vi "Problem_01b.vi"() -> ()   [LabVIEW 2023]
uses:
  <vilib>/regexp/Match Regular Expression.xnode
panel:
  out "string array":string[](array[string])
  out "x = y?":bool[](array[boolean])
  out "Array 2":i32[](array[numeric])
  out "sum":i32
  out "Array":i32[](array[numeric])
  in  "Puzzle":string="9cbncbxclbvkmfzdnldc\njjn1drdffhs\n3six7\n38rgtnqqxtc\nrxszdkkv3j8kjhbm\n54nzzddht8ninelrkkseightseven6\n6fourmnvkgnthjtnjqkr\nnineninezsstmkone4sjnlbldcrj4eight\n3rdnfkvrx4twoqgeightqkgmn\n6mlhponeglrzrvbsseven\nfive8spgxz8\n3three2dfourfour58\n9q\ntwo45\nfive8mpkpdfiveeightfourseven\n93threefive3three92\n6jdzeightnineone1sclhzrnrjxfive\n6nseven16lbztpbbzthree8five\neight6mntljvbfrmftsffchsix4\n4twosixvnhjl\n8d\neightsevenvqvzlqxkbm6rqhsgqpnine7twonex\nseven96\nck8tv6\n2mcddqpnbxssmrc6\nzsfbkrjjqpbbone6six2\nfourone8hfrkxrr\n7ninetphdpcx\n9gcn9six4mfnjgtcdc\n6onevsevenseven4three\nldssggpknine7\ntwolltbfkhltwo892jngx\nrsh1f..."
  in  "Sample":string="two1nine\neightwothree\nabcone2threexyz\nxtwone3four\n4nineeightseven2\nzoneight234\n7pqrstsixteen"
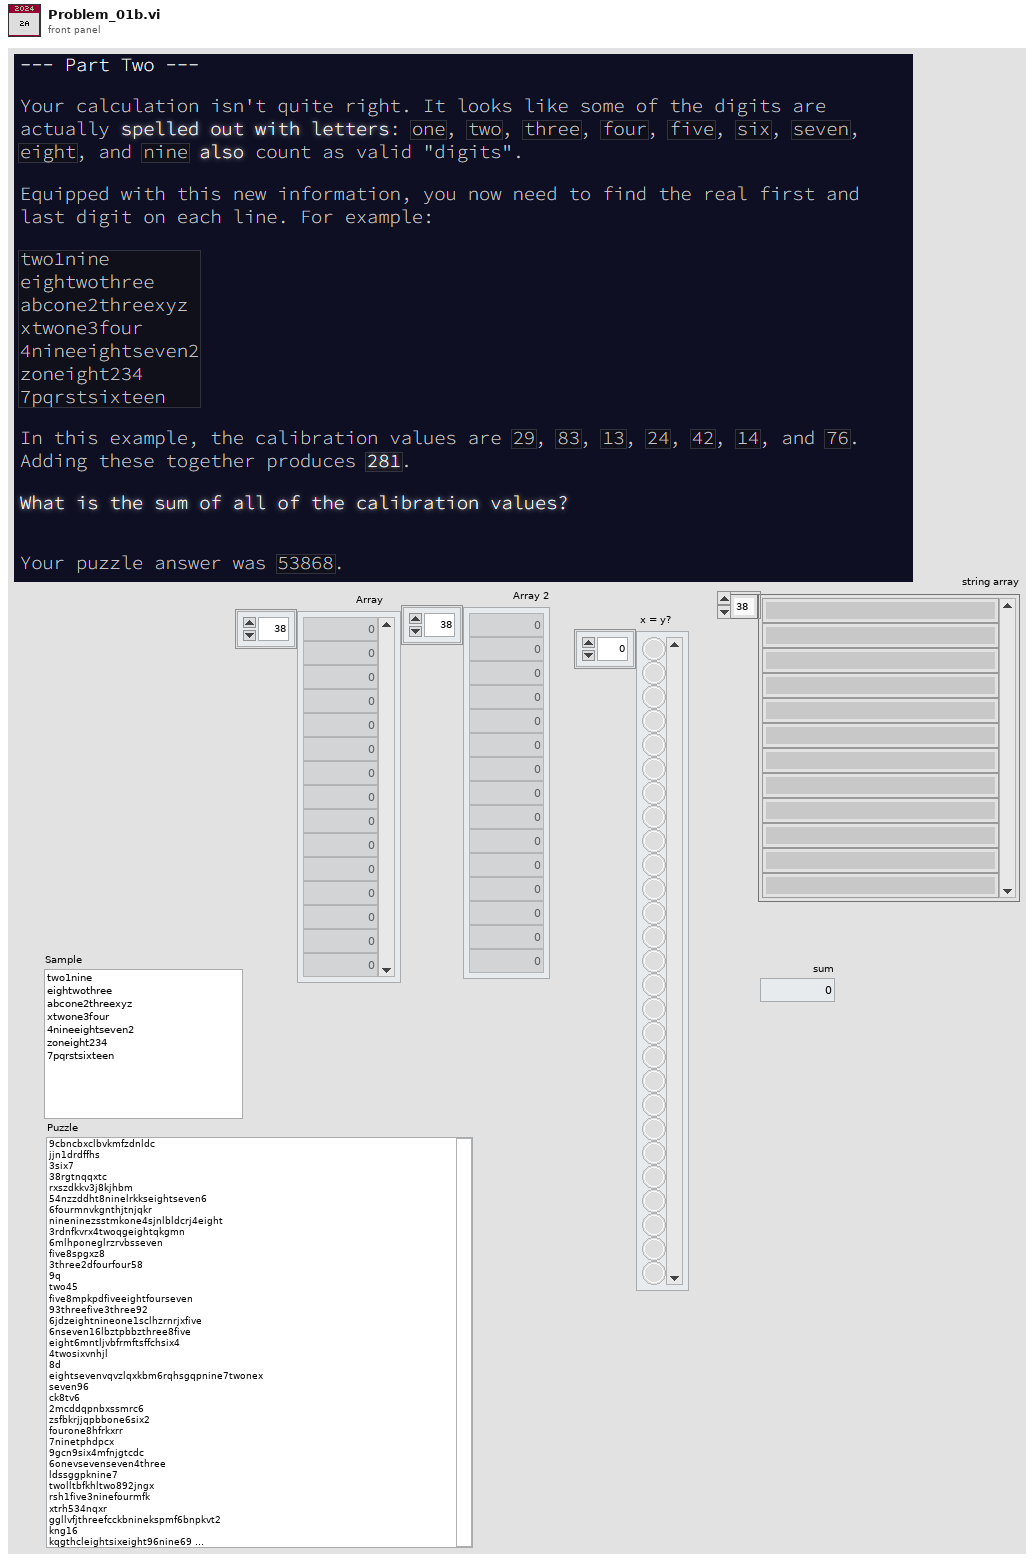
[diagram p1: front panel]
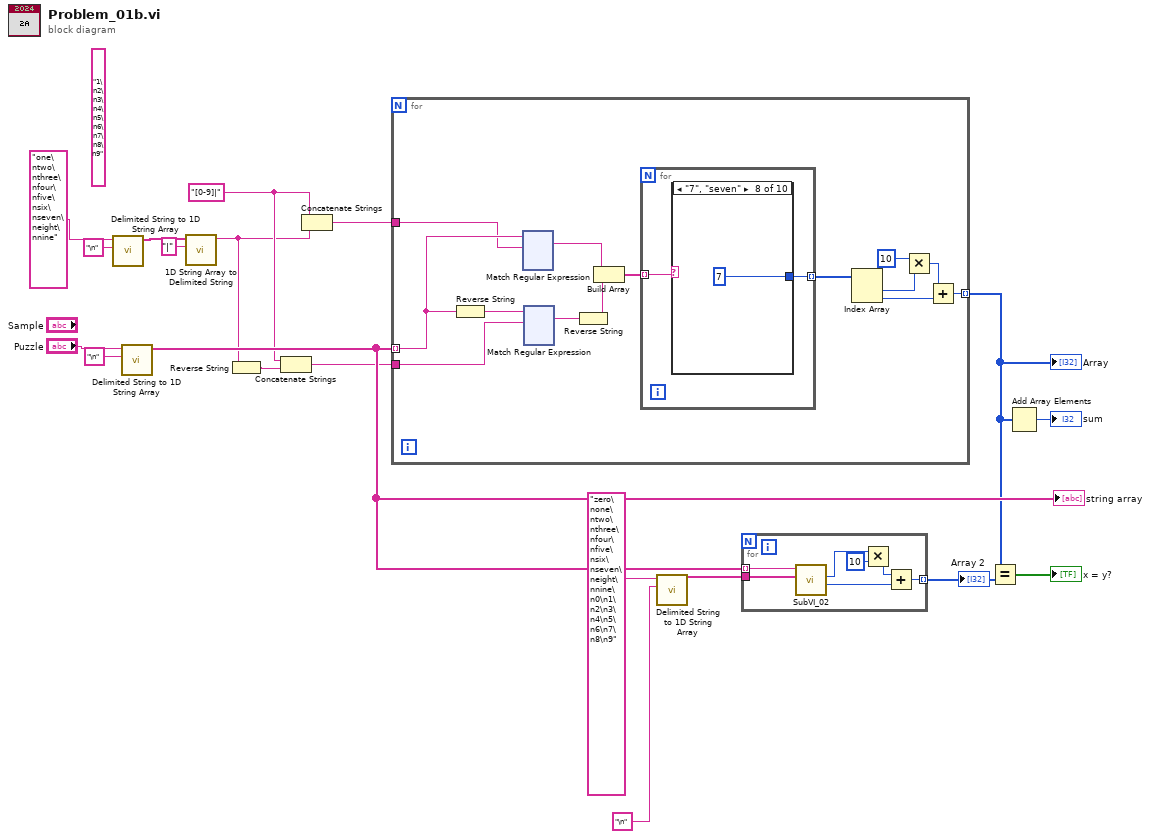
[diagram p0: block diagram]
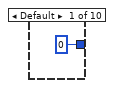
[diagram p2: hidden frame]
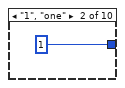
[diagram p3: hidden frame]
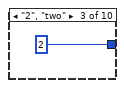
[diagram p4: hidden frame]
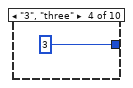
[diagram p5: hidden frame]
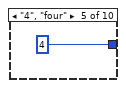
[diagram p6: hidden frame]
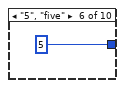
[diagram p7: hidden frame]
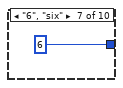
[diagram p8: hidden frame]
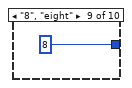
[diagram p9: hidden frame]
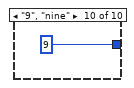
[diagram p10: hidden frame]
diagram:
  w4 = "[0-9]|" ("delimiter")
  (unwired) "1\n2\n3\n4\n5\n6\n7\n8\n9"
  n1 = call <vilib>:"Delimited String to 1D String Array.vi"("delimiter"="\n", "delimited string"="one\ntwo\nthree\nfour\nfive\nsix\nseven\neight\nnine") -> ("string array"=w14:string[])  [unwired: 9 in]
  n2 = call <vilib>:"Delimited String to 1D String Array.vi"("delimiter"="\n", "delimited string"="Puzzle") -> ("string array"=w13:string[])  [unwired: 9 in]
  "string array" <- w13
  n3 = call <vilib>:"1D String Array to Delimited String.vi"("delimiter"="|", "string array"=w14) -> ("delimited string"=w3:string)  [unwired: 9 in]
  n4 = Reverse String(1:w3) -> (0:w2:string)
  n5 = Concatenate Strings(w4, w2) -> (w1:string)
  n6 = Concatenate Strings(w4, w3) -> (w5:string)
  n7 = for {
    tunnel: w13 -> [w33] mode=indexing
    tunnel: w5 -> [w31]
    tunnel: w1 -> [w29]
    tunnel: [w20] -> w12 mode=indexing
    n8 = Reverse String(1:w33) -> (0:w32:string)
    n9 = xnode "Match Regular Expression"("input string"=w33, "regular expression"=w31) -> ("whole match"=w27:string)  [unwired: 4 in, 4 out]
    n10 = xnode "Match Regular Expression"("input string"=w32, "regular expression"=w29) -> ("whole match"=w30:string)  [unwired: 4 in, 4 out]
    n11 = Reverse String(1:w30) -> (0:w28:string)
    n12 = Build Array(w27, w28) -> (w26:string[])
    n13 = for {
      tunnel: w26 -> [w35] mode=indexing
      tunnel: [w34] -> w25 mode=indexing
      n14 = case shown="\"7\", \"seven\"" w35 {
        tunnel: [0 ("sum") 1 ("sum") 2 ("sum") 3 ("sum") 4 ("sum") 5 ("sum") 6 ("sum") 7 ("sum") 8 ("sum") 9 ("sum")] -> w34
        frame Default {
        }
        frame "1", "one" {
        }
        frame "2", "two" {
        }
        frame "3", "three" {
        }
        frame "4", "four" {
        }
        frame "5", "five" {
        }
        frame "6", "six" {
        }
        frame "7", "seven" {
        }
        frame "8", "eight" {
        }
        frame "9", "nine" {
        }
      }
    }
    n15 = Index Array(array=w25) -> (element #1=w24:i32, element #2=w21:i32)  [unwired: 2 in]
    n16 = Multiply(x=10, y=w24) -> (x*y=w22:i32)
    n17 = Add(x=w22, y=w21) -> (x+y=w20:i32)
  }
  "Array" <- w12
  n18 = call <vilib>:"Delimited String to 1D String Array.vi"("delimiter"="\n", "delimited string"="zero\none\ntwo\nthree\nfour\nfive\nsix\nseven\neight\nnine\n0\n1\n2\n3\n4\n5\n6\n7\n8\n9") -> ("string array"=w7:string[])  [unwired: 9 in]
  n19 = for {
    tunnel: w13 -> [w282] mode=indexing
    tunnel: [w283] -> w11 mode=indexing
    tunnel: w7 -> [w286]
    n20 = call "SubVI_02.vi"("string array"=w286, "String"=w282) -> ("Last"=w280:i32, "First"=w281:i32)  [unwired: 7 in, 1 out]
    n21 = Multiply(x=w281, y=10) -> (x*y=w284:i32)
    n22 = Add(x=w284, y=w280) -> (x+y=w283:i32)
  }
  "Array 2" <- w11
  n23 = Equal?(x=w12, y=w11) -> (x = y?=→"x = y?":bool[])
  n24 = Add Array Elements(numeric array=w12) -> (sum=→"sum":i32)
